vi "Delta_RT_manual_for_bigcryo.vi"() -> ()   [LabVIEW 2019]
uses:
  <vilib>/ptbypt/NI_PtbyPt.lvlib
panel:
  in  "Save R-H":bool
  in  "Measure R-H":bool
  in  "period [s]":dbl=0.5 caption="Delay Time (s)"
  out "R-H":cluster{"X":dbl[], "Y":dbl[]}[](graph) caption="XY Graph"
  in  "Reset R-H":bool
  in  "Period [s]":dbl=0.5 caption="Delay Time (s)"
  in  "Measure R-T":bool
  in  "Save R-T":bool
  out "R-T":cluster{"X":dbl[], "Y":dbl[]}[](graph) caption="XY Graph"
  out "Rate [K/min]":dbl=-0.03728307742891238 format="%#_6f"
  in  "Reset R-T":bool
  in  "Pause off":bool
  in  "Compliance [V]":dbl=1.0 format="%#_6f"
  out "VTI [K]":dbl=5.0082
  out "Delta Reading [Ohm]":dbl=1.19099581
  out "Sample Temp [K]":dbl=4.9552
  in  "Abort Delta":bool
  in  "Arm Delta":bool
  in  "DELAY [sec]":dbl=0.002 format="%#_6e"
  in  "I-HIGH [A]":dbl=0.0001 format="%#_6e"
  in  "Rate [K/min]":dbl=10.0
  in  "Set Temp [K]":dbl=1.0
  in  "Set Temperature":bool
  out "Magnetic Field [T]":dbl=-0.19938
  in  "Rate [T/min]":dbl=0.5
  in  "Set Field [T]":dbl=-0.2
  in  "Set Field":bool
  in  "Keithley":refnum<visa-resource-name>="GPIB1::20::INSTR"
  in  "Magnet Power supply":refnum<visa-resource-name>="COM7"
  in  "LakeShore350":refnum<visa-resource-name>="GPIB1::4::INSTR"
  out "error out 2":errorcluster={"status"=FALSE, "code"=1073676294, "source"="VISA Read in Delta_RT_manual_for_bigcryo.vi"}
  out "error out":errorcluster={"status"=FALSE, "code"=1073676294, "source"="VISA Read in Delta_RT_manual_for_bigcryo.vi"}
  # "Delta measurement"
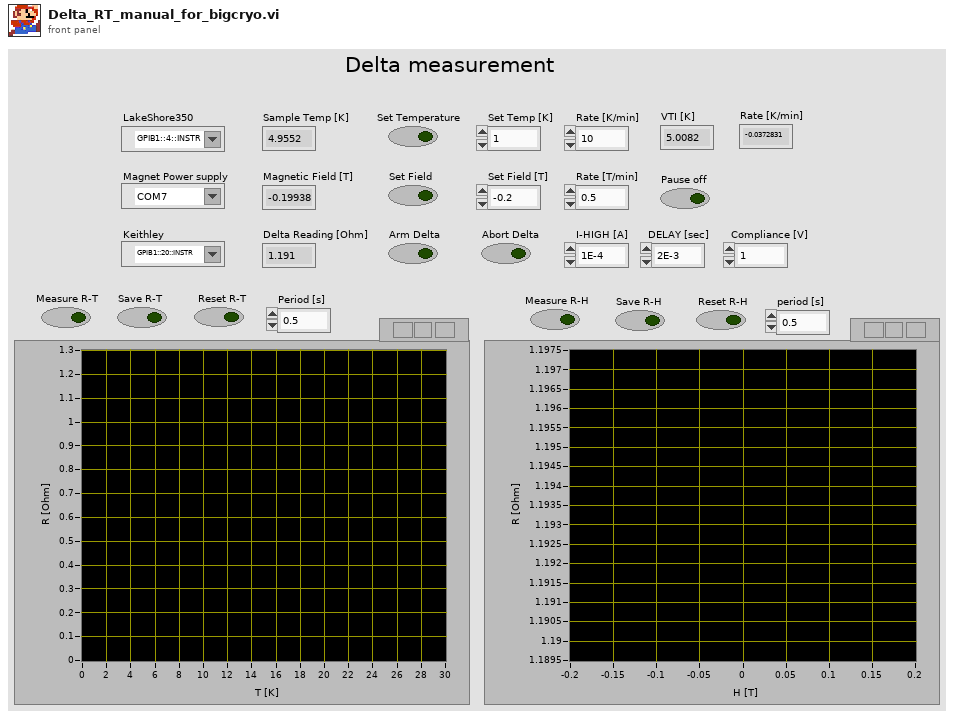
[diagram p1: front panel]
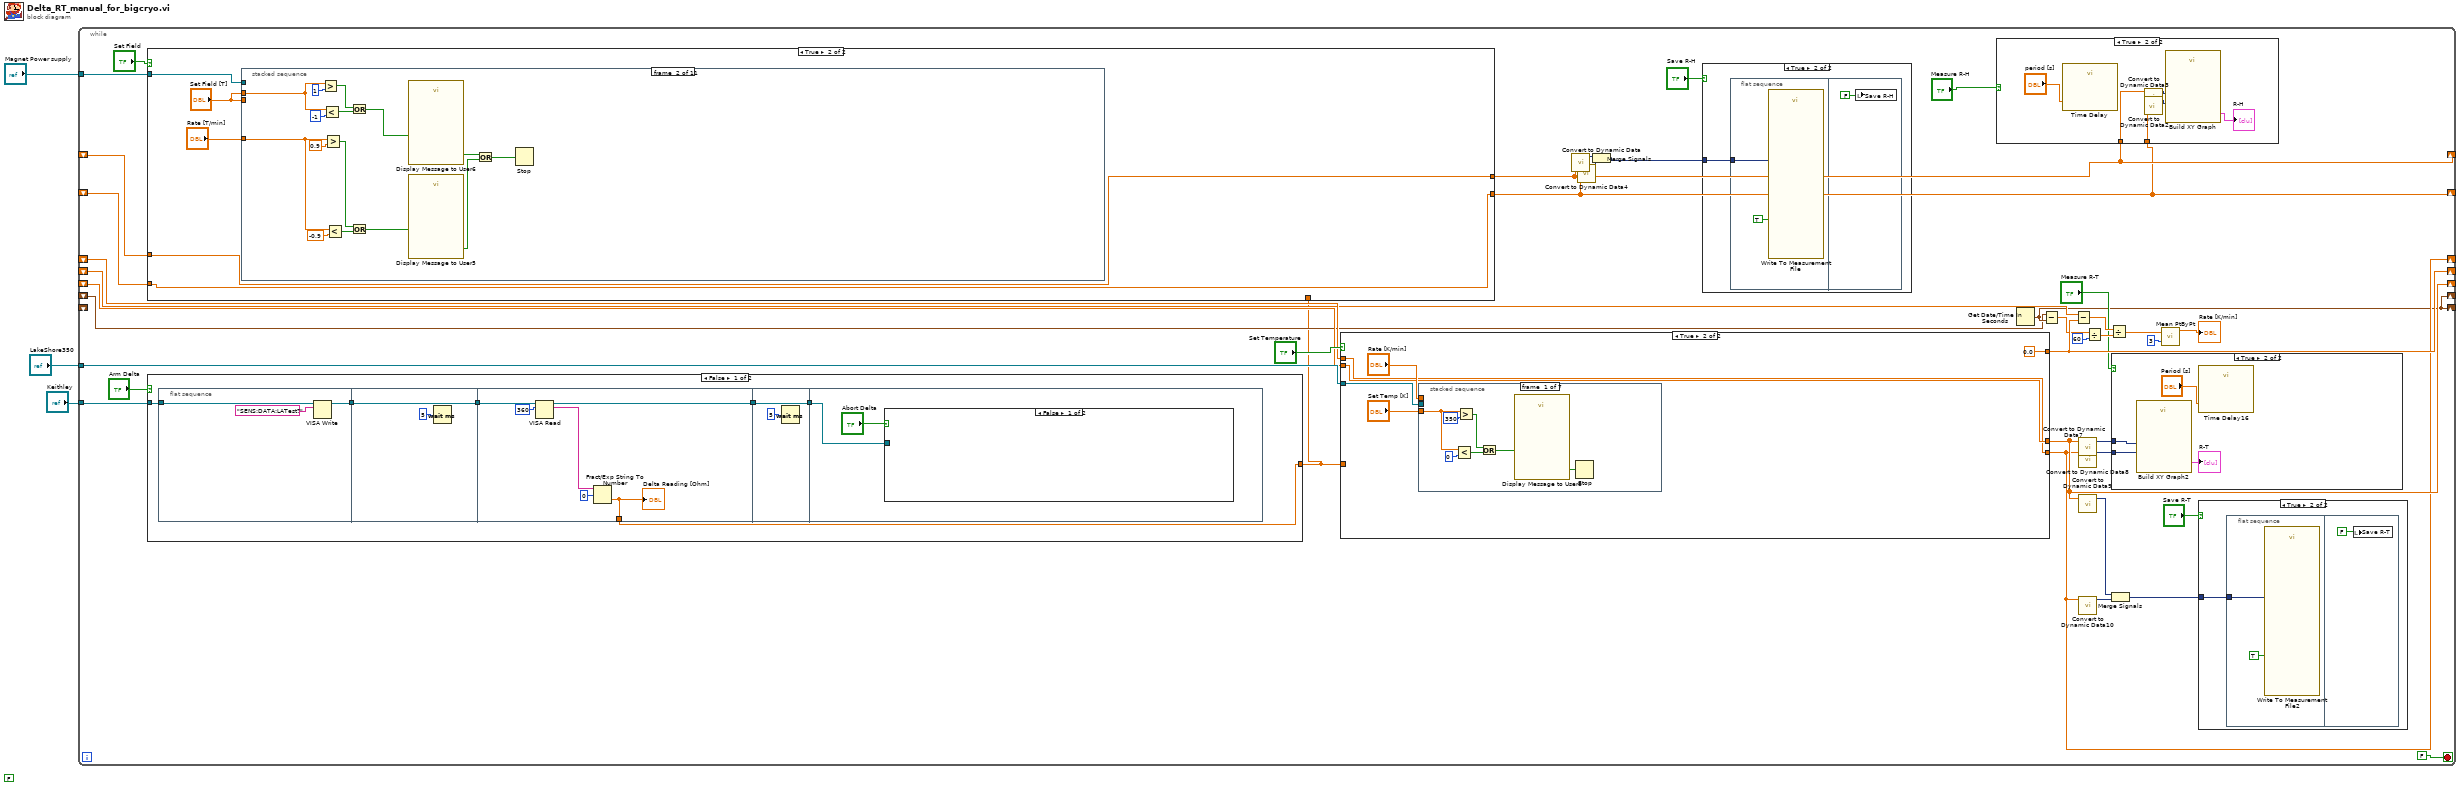
[diagram p0: block diagram]
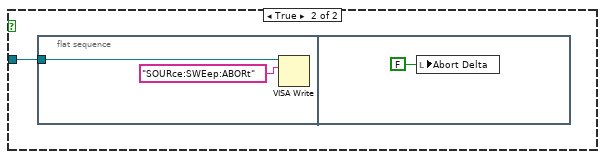
[diagram p6: hidden frame]
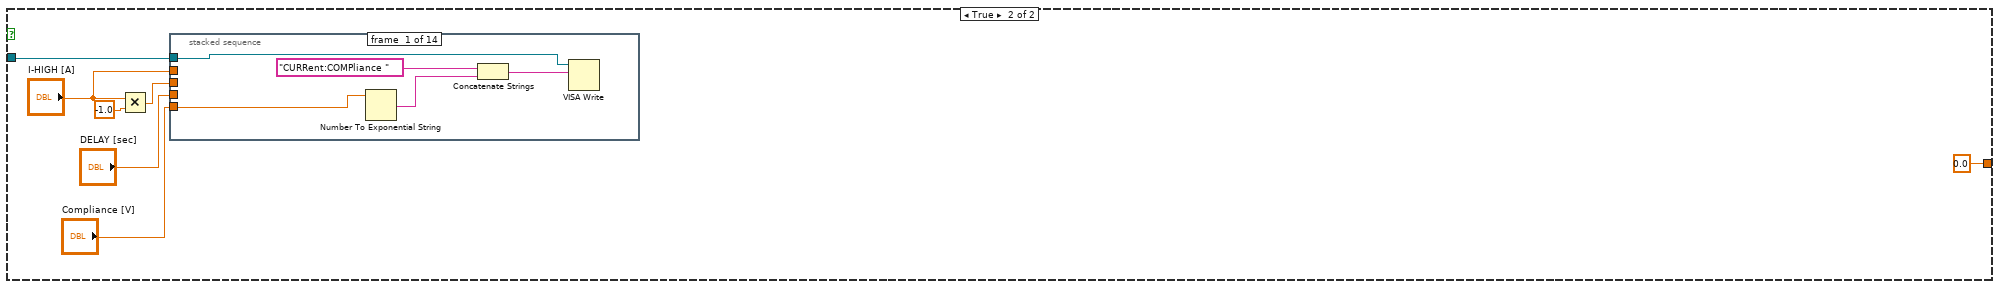
[diagram p7: hidden frame]
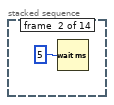
[diagram p8: hidden frame]
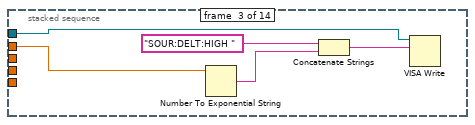
[diagram p9: hidden frame]
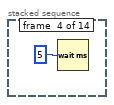
[diagram p10: hidden frame]
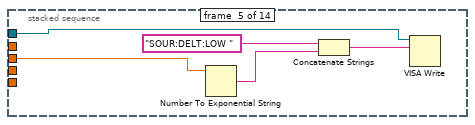
[diagram p11: hidden frame]
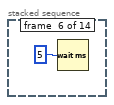
[diagram p12: hidden frame]
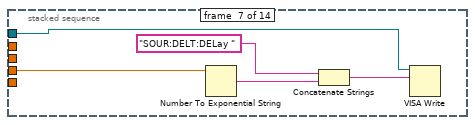
[diagram p13: hidden frame]
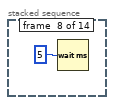
[diagram p14: hidden frame]
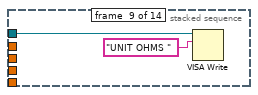
[diagram p15: hidden frame]
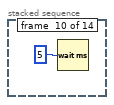
[diagram p16: hidden frame]
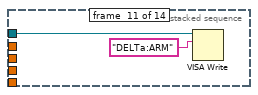
[diagram p17: hidden frame]
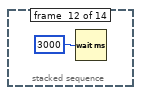
[diagram p18: hidden frame]
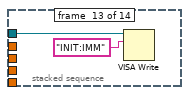
[diagram p19: hidden frame]
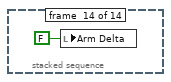
[diagram p20: hidden frame]
diagram:
  (unwired) FALSE
  n1 = while {
    tunnel: "Magnet Power supply" -> [w37]
    tunnel: "LakeShore350" -> [w40]
    tunnel: "Keithley" -> [w39]
    shift-right: [w26] -> _
    shift-left: _ -> [w21]
    shift-right: [w24] -> _
    shift-left: _ -> [w36]
    shift-right: [w19] -> _
    shift-left: _ -> [_]
    shift-right: [w34] -> _
    shift-left: _ -> [w35]
    shift-right: [w19] -> _
    shift-left: _ -> [w18]
    shift-right: [w7] -> _
    shift-left: _ -> [w12]
    shift-right: [w5] -> _
    shift-left: _ -> [w11]
    stop <- FALSE stop-if-true
    n2 = case shown="False" "Arm Delta" {
      tunnel: w39 -> [w66 w90]
      tunnel: [w61 0.0] -> w13
      frame False {
        n3 = flat-sequence {
          tunnel: w66 -> [w69]
          tunnel: [w67] -> w64
          tunnel: [w70] -> w65
          tunnel: w64 -> [w70]
          tunnel: w65 -> [w74]
          tunnel: [w73] -> w62
          tunnel: [w72] -> w61
          tunnel: [w78] -> w63
          tunnel: w62 -> [w78]
          tunnel: w63 -> [w80]
          frame #0 {
            n4 = VISA Write(VISA resource name=w69, write buffer="SENS:DATA:LATest?" ("write buffer 2")) -> (VISA resource name out=w67:refnum<visa-resource-name>)  [unwired: 1 in, 2 out]
          }
          frame #1 {
            n5 = Wait (ms)(milliseconds to wait=5) -> ()  [unwired: 1 out]
          }
          frame #2 {
            n6 = VISA Read(VISA resource name=w74, byte count=u32 360) -> (VISA resource name out=w73:refnum<visa-resource-name>, read buffer=w76:string)  [unwired: 1 in, 2 out]
            n7 = Fract/Exp String To Number(string=w76, offset=0) -> (number=w72:dbl)  [unwired: 3 out]
            "Delta Reading [Ohm]" <- w72
          }
          frame #3 {
            n8 = Wait (ms)(milliseconds to wait=5) -> ()  [unwired: 1 out]
          }
          frame #4 {
            n9 = case shown="False" "Abort Delta" {
              tunnel: w80 -> [_ w82]
              frame False {
              }
              frame True {
                n10 = flat-sequence {
                  tunnel: w82 -> [w84]
                  frame #0 {
                    n11 = VISA Write(VISA resource name=w84, write buffer="SOURce:SWEep:ABORt") -> ()  [unwired: 1 in, 3 out]
                  }
                  frame #1 {
                    n12 = local write "Abort Delta"(FALSE) -> ()
                  }
                }
              }
            }
          }
        }
      }
      frame True {
        n13 = Multiply(x="I-HIGH [A]", y=-1.0) -> (x*y=w89:dbl)
        n14 = stacked-sequence {
          tunnel: "I-HIGH [A]" -> [_ _ w101 _ _ _ _ _ _ _ _ _ _ _]
          tunnel: w90 -> [w94 _ w99 _ w106 _ w112 _ w117 _ w120 _ w123 _]
          tunnel: w89 -> [_ _ _ _ w105 _ _ _ _ _ _ _ _ _]
          tunnel: "DELAY [sec]" -> [_ _ _ _ _ _ w111 _ _ _ _ _ _ _]
          tunnel: "Compliance [V]" -> [w93 _ _ _ _ _ _ _ _ _ _ _ _ _]
          frame #0 {
            n15 = Number To Exponential String(number=w93) -> (E-format string=w96:string)  [unwired: 3 in]
            n16 = Concatenate Strings("CURRent:COMPliance ", w96) -> (w95:string)
            n17 = VISA Write(VISA resource name=w94, write buffer=w95) -> ()  [unwired: 1 in, 3 out]
          }
          frame #1 {
            n18 = Wait (ms)(milliseconds to wait=5) -> ()  [unwired: 1 out]
          }
          frame #2 {
            n19 = Number To Exponential String(number=w101) -> (E-format string=w102:string)  [unwired: 3 in]
            n20 = Concatenate Strings("SOUR:DELT:HIGH ", w102) -> (w100:string)
            n21 = VISA Write(VISA resource name=w99, write buffer=w100) -> ()  [unwired: 1 in, 3 out]
          }
          frame #3 {
            n22 = Wait (ms)(milliseconds to wait=5) -> ()  [unwired: 1 out]
          }
          frame #4 {
            n23 = Number To Exponential String(number=w105) -> (E-format string=w108:string)  [unwired: 3 in]
            n24 = Concatenate Strings("SOUR:DELT:LOW ", w108) -> (w107:string)
            n25 = VISA Write(VISA resource name=w106, write buffer=w107) -> ()  [unwired: 1 in, 3 out]
          }
          frame #5 {
            n26 = Wait (ms)(milliseconds to wait=5) -> ()  [unwired: 1 out]
          }
          frame #6 {
            n27 = Number To Exponential String(number=w111) -> (E-format string=w114:string)  [unwired: 3 in]
            n28 = Concatenate Strings("SOUR:DELT:DELay ", w114) -> (w113:string)
            n29 = VISA Write(VISA resource name=w112, write buffer=w113) -> ()  [unwired: 1 in, 3 out]
          }
          frame #7 {
            n30 = Wait (ms)(milliseconds to wait=5) -> ()  [unwired: 1 out]
          }
          frame #8 {
            n31 = VISA Write(VISA resource name=w117, write buffer="UNIT OHMS ") -> ()  [unwired: 1 in, 3 out]
          }
          frame #9 {
            n32 = Wait (ms)(milliseconds to wait=5) -> ()  [unwired: 1 out]
          }
          frame #10 {
            n33 = VISA Write(VISA resource name=w120, write buffer="DELTa:ARM") -> ()  [unwired: 1 in, 3 out]
          }
          frame #11 {
            n34 = Wait (ms)(milliseconds to wait=3000) -> ()  [unwired: 1 out]
          }
          frame #12 {
            n35 = VISA Write(VISA resource name=w123, write buffer="INIT:IMM") -> ()  [unwired: 1 in, 3 out]
          }
          frame #13 {
            n36 = local write "Arm Delta"(FALSE) -> ()
          }
        }
      }
    }
    n37 = case shown="True" "Set Field" {
      tunnel: w37 -> [w206 w289]
      tunnel: w13 -> [w204 _]
      tunnel: [w203 w288] -> w7
      tunnel: w12 -> [w202 w288]
      tunnel: [w201 w287] -> w5
      tunnel: w11 -> [w200 w287]
      frame False {
        n38 = stacked-sequence {
          seq-local: [w218 _ _ _ _ _ _ _] -> [_ w221 _ _ _ _ _ _]
          seq-local: [_ w219 _ _ _ _ _ _] -> [_ _ w225 _ _ _ _ _]
          seq-local: [_ w220 _ _ _ _ _ _] -> [_ _ w222 _ _ _ _ _]
          seq-local: [_ _ w224 _ _ _ _ _] -> [_ _ _ w265 _ _ _ _]
          seq-local: [_ _ w223 _ _ _ _ _] -> [_ _ _ w264 _ _ _ _]
          seq-local: [_ _ _ w267 _ _ _ _] -> [_ _ _ _ w270 _ _ _]
          seq-local: [_ _ _ w266 _ _ _ _] -> [_ _ _ _ w271 _ _ _]
          seq-local: [_ _ _ _ w270 _ _ _] -> [_ _ _ _ _ w282 _ _]
          seq-local: [_ _ _ _ w271 _ _ _] -> [_ _ _ _ _ w280 _ _]
          seq-local: [_ _ _ _ _ w281 _ _] -> [_ _ _ _ _ _ _ w286]
          seq-local: [_ _ _ _ _ w279 _ _] -> [_ _ _ _ _ _ _ w285]
          tunnel: w206 -> [w218 _ _ _ _ _ _ _]
          tunnel: [_ _ _ _ _ w272 _ _] -> w205
          frame #0 {
          }
          frame #1 {
            n39 = VISA Clear(VISA resource name=w221) -> (VISA resource name out=w219:refnum<visa-resource-name>, error out=w220:errorcluster)  [unwired: 1 in]
          }
          frame #2 {
            n40 = flat-sequence {
              tunnel: w225 -> [w229]
              tunnel: [w228] -> w224
              tunnel: [w227] -> w223
              tunnel: w222 -> [w226]
              frame #0 {
                n41 = call "Time Delay8"() -> ()  [unwired: 11 in, 1 out]
              }
              frame #1 {
                n42 = case shown="False" "Pause off" {
                  tunnel: w229 -> [w232 w244]
                  tunnel: [w232 w233] -> w228
                  tunnel: [w231 w236] -> w227
                  tunnel: w226 -> [w231 w239]
                  frame False {
                  }
                  frame True {
                    n43 = flat-sequence {
                      tunnel: w244 -> [w248]
                      tunnel: [w247] -> w242
                      tunnel: [w246] -> w240
                      tunnel: w239 -> [w245]
                      tunnel: [w253] -> w243
                      tunnel: w242 -> [w253]
                      tunnel: [w252] -> w241
                      tunnel: w240 -> [w252]
                      tunnel: w243 -> [w255]
                      tunnel: w241 -> [_]
                      tunnel: [w255] -> w238
                      tunnel: [w254] -> w234
                      tunnel: w238 -> [w257]
                      tunnel: [w257] -> w237
                      tunnel: [w256] -> w235
                      tunnel: w234 -> [w256]
                      tunnel: [w261] -> w233
                      tunnel: w237 -> [w260]
                      tunnel: [w259] -> w236
                      tunnel: w235 -> [w258]
                      frame #0 {
                        n44 = Concatenate Strings("P 0" ("Command"), "\r") -> (w250:string)
                        n45 = VISA Write(VISA resource name=w248, write buffer=w250, error in (no error)=w245) -> (VISA resource name out=w247:refnum<visa-resource-name>, error out=w246:errorcluster)  [unwired: 1 out]
                      }
                      frame #1 {
                        n46 = call "Time Delay14"() -> ()  [unwired: 11 in, 1 out]
                      }
                      frame #2 {
                        n47 = VISA Close(VISA resource name=w255) -> (error out=w254:errorcluster)  [unwired: 1 in]
                      }
                      frame #3 {
                        n48 = call "Time Delay15"() -> ()  [unwired: 11 in, 1 out]
                      }
                      frame #4 {
                        n49 = VISA Clear(VISA resource name=w260, error in (no error)=w258) -> (VISA resource name out=w261:refnum<visa-resource-name>, error out=w259:errorcluster)
                      }
                      frame #5 {
                        n50 = local write "Pause off"(FALSE) -> ()
                      }
                    }
                  }
                }
              }
            }
          }
          frame #3 {
            n51 = Concatenate Strings("G O" ("Command"), "\r") -> (w268:string)
            n52 = VISA Write(VISA resource name=w265, write buffer=w268, error in (no error)=w264) -> (VISA resource name out=w267:refnum<visa-resource-name>, error out=w266:errorcluster)  [unwired: 1 out]
          }
          frame #4 {
            n53 = call "Time Delay9"() -> ()  [unwired: 11 in, 1 out]
          }
          frame #5 {
            n54 = VISA Read(VISA resource name=w282, byte count=u32 30, error in (no error)=w280) -> (VISA resource name out=w281:refnum<visa-resource-name>, read buffer=w276:string, error out=w279:errorcluster)  [unwired: 1 out]
            n55 = Match Pattern(string=w276, regular expression="OUTPUT:") -> (after substring=w274:string)  [unwired: 1 in, 3 out]
            n56 = Match Pattern(string=w274, regular expression=" TESLA") -> (before substring=w273:string)  [unwired: 1 in, 3 out]
            n57 = Fract/Exp String To Number(string=w273, offset=0) -> (number=w272:dbl)  [unwired: 2 in, 1 out]
          }
          frame #6 {
            n58 = call "Time Delay10"() -> ()  [unwired: 11 in, 1 out]
          }
          frame #7 {
            n59 = VISA Close(VISA resource name=w286, error in (no error)=w285) -> (error out=→"error out":errorcluster)
          }
        }
        "Magnetic Field [T]" <- w205
        n60 = case shown="False" "Reset R-H" {
          tunnel: w205 -> [w212 _]
          tunnel: [w211 w214] -> w203
          tunnel: [w210 w213] -> w201
          tunnel: w204 -> [w209 _]
          tunnel: w202 -> [w208 _]
          tunnel: w200 -> [w207 _]
          frame False {
            n61 = Build Array (concatenate)(w208, w212) -> (w211:dbl[])
            n62 = Build Array (concatenate)(w207, w209) -> (w210:dbl[])
          }
          frame True {
            n63 = stacked-sequence {
              tunnel: [dbl[] [] _] -> w214
              tunnel: [dbl[] [] _] -> w213
              frame #0 {
              }
              frame #1 {
                n64 = local write "Reset R-H"(FALSE) -> ()
              }
            }
          }
        }
      }
      frame True {
        n65 = stacked-sequence {
          tunnel: w289 -> [w292 _ _ w311 _ w356 _ w374 _ w379 _]
          tunnel: "Set Field [T]" -> [_ w294 _ _ _ _ _ _ _ _ _]
          tunnel: "Rate [T/min]" -> [_ w293 _ _ _ _ _ w364 _ _ _]
          tunnel: "Set Field [T]" -> [_ _ _ w310 _ w354 _ _ _ _ _]
          frame #0 {
            n66 = VISA Clear(VISA resource name=w292) -> ()  [unwired: 1 in, 2 out]
          }
          frame #1 {
            n67 = Greater?(x=w294, y=1) -> (0:w295:bool)
            n68 = Less?(x=w294, y=-1) -> (x < y?=w300:bool)
            n69 = Greater?(x=w293, y=0.9) -> (0:w304:bool)
            n70 = Less?(x=w293, y=-0.9) -> (x < y?=w303:bool)
            n71 = Or(x=w295, y=w300) -> (x .or. y?=w306:bool)
            n72 = Or(x=w304, y=w303) -> (x .or. y?=w305:bool)
            n73 = call "Display Message to User6"("Enable"=w306) -> ("OK"=w307:bool)  [unwired: 9 in, 1 out]
            n74 = call "Display Message to User5"("Enable"=w305) -> ("OK"=w296:bool)  [unwired: 9 in, 1 out]
            n75 = Or(x=w307, y=w296) -> (x .or. y?=w297:bool)
            n76 = Stop(stop? (T)=w297) -> ()
          }
          frame #2 {
            n77 = Wait (ms)(milliseconds to wait=500) -> ()  [unwired: 1 out]
          }
          frame #3 {
            # "Read Magnetic Field"
            # "for safety"
            # "polarity"
            n78 = stacked-sequence {
              seq-local: [w315 _ _ _ _ _ _ _] -> [_ w318 _ _ _ _ _ _]
              seq-local: [_ w316 _ _ _ _ _ _] -> [_ _ w320 _ _ _ _ _]
              seq-local: [_ w317 _ _ _ _ _ _] -> [_ _ w319 _ _ _ _ _]
              seq-local: [_ _ w320 _ _ _ _ _] -> [_ _ _ w323 _ _ _ _]
              seq-local: [_ _ w319 _ _ _ _ _] -> [_ _ _ w322 _ _ _ _]
              seq-local: [_ _ _ w325 _ _ _ _] -> [_ _ _ _ w328 _ _ _]
              seq-local: [_ _ _ w324 _ _ _ _] -> [_ _ _ _ w329 _ _ _]
              seq-local: [_ _ _ _ w328 _ _ _] -> [_ _ _ _ _ w340 _ _]
              seq-local: [_ _ _ _ w329 _ _ _] -> [_ _ _ _ _ w338 _ _]
              seq-local: [_ _ _ _ _ w339 _ _] -> [_ _ _ _ _ _ _ w344]
              seq-local: [_ _ _ _ _ w337 _ _] -> [_ _ _ _ _ _ _ w343]
              tunnel: w311 -> [w315 _ _ _ _ _ _ _]
              tunnel: [_ _ _ _ _ w330 _ _] -> w312
              frame #0 {
              }
              frame #1 {
                n79 = VISA Clear(VISA resource name=w318) -> (VISA resource name out=w316:refnum<visa-resource-name>, error out=w317:errorcluster)  [unwired: 1 in]
              }
              frame #2 {
                n80 = call "Time Delay6"() -> ()  [unwired: 11 in, 1 out]
              }
              frame #3 {
                n81 = Concatenate Strings("G O" ("Command"), "\r") -> (w326:string)
                n82 = VISA Write(VISA resource name=w323, write buffer=w326, error in (no error)=w322) -> (VISA resource name out=w325:refnum<visa-resource-name>, error out=w324:errorcluster)  [unwired: 1 out]
              }
              frame #4 {
                n83 = call "Time Delay7"() -> ()  [unwired: 11 in, 1 out]
              }
              frame #5 {
                n84 = VISA Read(VISA resource name=w340, byte count=u32 30, error in (no error)=w338) -> (VISA resource name out=w339:refnum<visa-resource-name>, read buffer=w334:string, error out=w337:errorcluster)  [unwired: 1 out]
                n85 = Match Pattern(string=w334, regular expression="OUTPUT:") -> (after substring=w332:string)  [unwired: 1 in, 3 out]
                n86 = Match Pattern(string=w332, regular expression=" TESLA") -> (before substring=w331:string)  [unwired: 1 in, 3 out]
                n87 = Fract/Exp String To Number(string=w331, offset=0) -> (number=w330:dbl)  [unwired: 2 in, 1 out]
              }
              frame #6 {
                n88 = call "Time Delay11"() -> ()  [unwired: 11 in, 1 out]
              }
              frame #7 {
                n89 = VISA Close(VISA resource name=w344, error in (no error)=w343) -> (error out=→"error out 2":errorcluster)
              }
            }
            n90 = Absolute Value(x=w312) -> (abs(x)=w313:dbl)
            n91 = Less?(x=w313, y=0.002) -> (x < y?=w309:bool)
            n92 = case shown="True" w309 {
              tunnel: w311 -> [_ w347]
              tunnel: w310 -> [_ w345]
              frame False {
              }
              frame True {
                n93 = Greater Or Equal To 0?(x=w345) -> (x >= 0?=w346:bool)
                n94 = case shown="True" w346 {
                  tunnel: ["D [-]" ("data") "D [+]" ("data")] -> w348
                  frame False {
                  }
                  frame True {
                  }
                }
                n95 = Concatenate Strings(w348, "\r") -> (w350:string)
                n96 = VISA Write(VISA resource name=w347, write buffer=w350) -> ()  [unwired: 1 in, 3 out]
              }
            }
          }
          frame #4 {
            n97 = Wait (ms)(milliseconds to wait=500) -> ()  [unwired: 1 out]
          }
          frame #5 {
            # "set set field"
            n98 = Number To Fractional String(number=w354, width (-)=i16 6, precision (6)=i16 3) -> (F-format string=w359:string)  [unwired: 1 in]
            n99 = Concatenate Strings("S [%][MID] " ("string"), w359) -> (w355:string)
            n100 = Concatenate Strings(w355, "\r") -> (w358:string)
            n101 = VISA Write(VISA resource name=w356, write buffer=w358) -> ()  [unwired: 1 in, 3 out]
          }
          frame #6 {
            n102 = Wait (ms)(milliseconds to wait=500) -> ()  [unwired: 1 out]
          }
          frame #7 {
            # "set rate"
            n103 = Divide(x=w364, y=60.0) -> (x/y=w369:dbl)
            n104 = Divide(x=w369, y=0.09797) -> (x/y=w367:dbl)
            n105 = Number To Fractional String(number=w367, width (-)=i16 6, precision (6)=i16 3) -> (F-format string=w372:string)  [unwired: 1 in]
            n106 = Concatenate Strings("S R " ("string"), w372) -> (w371:string)
            n107 = Concatenate Strings(w371, "\r") -> (w376:string)
            n108 = VISA Write(VISA resource name=w374, write buffer=w376) -> ()  [unwired: 1 in, 3 out]
          }
          frame #8 {
            n109 = Wait (ms)(milliseconds to wait=500) -> ()  [unwired: 1 out]
          }
          frame #9 {
            # "Go to set field"
            n110 = Concatenate Strings("R [%][MID]" ("data"), "\r") -> (w381:string)
            n111 = VISA Write(VISA resource name=w379, write buffer=w381) -> ()  [unwired: 1 in, 3 out]
          }
          frame #10 {
            n112 = local write "Set Field"(FALSE) -> ()
            n113 = Wait (ms)(milliseconds to wait=500) -> ()  [unwired: 1 out]
          }
        }
      }
    }
    n114 = case shown="True" "Set Temperature" {
      tunnel: w40 -> [w136 w172]
      tunnel: [w131 w169] -> w26
      tunnel: w21 -> [w132 w169]
      tunnel: w13 -> [w130 _]
      tunnel: [w129 w168] -> w24
      tunnel: w36 -> [w128 w168]
      tunnel: [w126 0.0] -> w34
      frame False {
        n115 = flat-sequence {
          tunnel: w136 -> [w150]
          tunnel: [w149] -> w134
          tunnel: [w148] -> w133
          tunnel: [w148] -> w126
          tunnel: [w157] -> w135
          tunnel: w134 -> [w157]
          tunnel: w135 -> [w159]
          frame #0 {
            n116 = Concatenate Strings("KRDG?B" ("write buffer"), "\n") -> (w155:string)
            n117 = VISA Write(VISA resource name=w150, write buffer=w155) -> (VISA resource name out=w153:refnum<visa-resource-name>)  [unwired: 1 in, 2 out]
            n118 = VISA Read(VISA resource name=w153, byte count=u32 100) -> (VISA resource name out=w149:refnum<visa-resource-name>, read buffer=w151:string)  [unwired: 1 in, 2 out]
            n119 = Fract/Exp String To Number(string=w151) -> (number=w148:dbl)  [unwired: 3 in, 1 out]
            "Sample Temp [K]" <- w148
          }
          frame #1 {
            n120 = Wait (ms)(milliseconds to wait=5) -> ()  [unwired: 1 out]
          }
          frame #2 {
            n121 = Concatenate Strings("KRDG?A" ("write buffer"), "\n") -> (w165:string)
            n122 = VISA Write(VISA resource name=w159, write buffer=w165) -> (VISA resource name out=w163:refnum<visa-resource-name>)  [unwired: 1 in, 2 out]
            n123 = VISA Read(VISA resource name=w163, byte count=u32 100) -> (read buffer=w161:string)  [unwired: 1 in, 3 out]
            n124 = Fract/Exp String To Number(string=w161) -> (number=→"VTI [K]":dbl)  [unwired: 3 in, 1 out]
          }
        }
        n125 = case shown="False" "Reset R-T" {
          tunnel: w133 -> [w142 _]
          tunnel: w132 -> [w141 _]
          tunnel: [w140 w144] -> w131
          tunnel: w130 -> [w139 _]
          tunnel: [w138 w143] -> w129
          tunnel: w128 -> [w137 _]
          frame False {
            n126 = Build Array (concatenate)(w141, w142) -> (w140:dbl[])
            n127 = Build Array (concatenate)(w137, w139) -> (w138:dbl[])
          }
          frame True {
            n128 = stacked-sequence {
              tunnel: [dbl[] [] _] -> w144
              tunnel: [dbl[] [] _] -> w143
              frame #0 {
              }
              frame #1 {
                n129 = local write "Reset R-T"(FALSE) -> ()
              }
            }
          }
        }
      }
      frame True {
        n130 = stacked-sequence {
          tunnel: w172 -> [_ w180 _ w187 _ w194 _]
          tunnel: "Set Temp [K]" -> [w174 _ _ _ _ w192 _]
          tunnel: "Rate [K/min]" -> [_ _ _ w186 _ _ _]
          frame #0 {
            n131 = Less?(x=w174, y=0) -> (x < y?=w178:bool)
            n132 = Greater?(x=w174, y=350) -> (0:w175:bool)
            n133 = Or(x=w175, y=w178) -> (x .or. y?=w179:bool)
            n134 = call "Display Message to User8"("Enable"=w179) -> ("OK"=w173:bool)  [unwired: 9 in, 1 out]
            n135 = Stop(stop? (T)=w173) -> ()
          }
          frame #1 {
            n136 = Concatenate Strings("OUTMODE 1, 1, 2, 1" ("write buffer"), "\n") -> (w181:string)
            n137 = VISA Write(VISA resource name=w180, write buffer=w181) -> ()  [unwired: 1 in, 3 out]
          }
          frame #2 {
            n138 = Wait (ms)(milliseconds to wait=u32 50) -> ()  [unwired: 1 out]
          }
          frame #3 {
            n139 = Number To Fractional String(number=w186) -> (F-format string=w185:string)  [unwired: 3 in]
            n140 = Concatenate Strings("RAMP 1, 1," ("write buffer"), w185, "\n") -> (w189:string)
            n141 = VISA Write(VISA resource name=w187, write buffer=w189) -> ()  [unwired: 1 in, 3 out]
          }
          frame #4 {
            n142 = Wait (ms)(milliseconds to wait=u32 50) -> ()  [unwired: 1 out]
          }
          frame #5 {
            n143 = Number To Fractional String(number=w192) -> (F-format string=w193:string)  [unwired: 3 in]
            n144 = Concatenate Strings("SETP 1," ("write buffer"), w193, "\n") -> (w196:string)
            n145 = VISA Write(VISA resource name=w194, write buffer=w196) -> ()  [unwired: 1 in, 3 out]
          }
          frame #6 {
            n146 = local write "Set Temperature"(FALSE) -> ()
          }
        }
      }
    }
    n147 = call "Convert to Dynamic Data"("Array"=w7) -> ("Dynamic Data Type"=w6:dynamicdata)  [unwired: 3 in]
    n148 = call "Convert to Dynamic Data4"("Array"=w5) -> ("Dynamic Data Type"=w4:dynamicdata)  [unwired: 3 in]
    n149 = Merge Signals(w6, w4) -> (w8:dynamicdata)
    n150 = case shown="True" "Save R-H" {
      tunnel: w8 -> [_ w43]
      frame False {
      }
      frame True {
        n151 = flat-sequence {
          tunnel: w43 -> [w44]
          frame #0 {
            n152 = call "Write To Measurement File"("Signals"=w44, "Reset"=TRUE) -> ()  [unwired: 15 in, 3 out]
          }
          frame #1 {
            n153 = local write "Save R-H"(FALSE) -> ()
          }
        }
      }
    }
    n154 = case shown="True" "Measure R-H" {
      tunnel: w5 -> [_ w51]
      tunnel: w7 -> [_ w49]
      frame False {
      }
      frame True {
        n155 = call "Time Delay"("Delay Time (s)"="period [s]") -> ()  [unwired: 10 in, 1 out]
        n156 = call "Convert to Dynamic Data3"("Array"=w49) -> ("Dynamic Data Type"=w48:dynamicdata)  [unwired: 3 in]
        n157 = call "Convert to Dynamic Data2"("Array"=w51) -> ("Dynamic Data Type"=w50:dynamicdata)  [unwired: 3 in]
        n158 = call "Build XY Graph"("Y Input"=w50, "X Input"=w48) -> ("XY Graph"=→"R-H":cluster{"X":dbl[], "Y":dbl[]}[])  [unwired: 8 in, 1 out]
      }
    }
    n159 = Get Date/Time In Seconds() -> (seconds since 1Jan1904=w19:timestamp)
    n160 = Subtract(x=w18, y=w19) -> (x-y=w33:dbl)
    n161 = Subtract(x=w35, y=w34) -> (x-y=w30:dbl)
    n162 = call "Convert to Dynamic Data7"("Array"=w26) -> ("Dynamic Data Type"=w29:dynamicdata)  [unwired: 3 in]
    n163 = call "Convert to Dynamic Data8"("Array"=w24) -> ("Dynamic Data Type"=w28:dynamicdata)  [unwired: 3 in]
    n164 = call "Convert to Dynamic Data9"("Array"=w26) -> ("Dynamic Data Type"=w25:dynamicdata)  [unwired: 3 in]
    n165 = call "Convert to Dynamic Data10"("Array"=w24) -> ("Dynamic Data Type"=w23:dynamicdata)  [unwired: 3 in]
    n166 = Divide(x=w33, y=60) -> (x/y=w31:dbl)
    n167 = Divide(x=w30, y=w31) -> (x/y=w16:dbl)
    n168 = case shown="True" "Measure R-T" {
      tunnel: w29 -> [_ w56]
      tunnel: w28 -> [_ w53]
      frame False {
      }
      frame True {
        n169 = call "Build XY Graph2"("Y Input"=w53, "X Input"=w56) -> ("XY Graph"=→"R-T":cluster{"X":dbl[], "Y":dbl[]}[])  [unwired: 8 in, 1 out]
        n170 = call "Time Delay16"("Delay Time (s)"="Period [s]") -> ()  [unwired: 10 in, 1 out]
      }
    }
    n171 = Merge Signals(w25, w23) -> (w27:dynamicdata)
    n172 = call <vilib>:"Mean PtByPt.vi"("x"=w16, "sample length"=3) -> ("mean"=→"Rate [K/min]":dbl)  [unwired: 2 in, 1 out]
    n173 = case shown="True" "Save R-T" {
      tunnel: w27 -> [_ w57]
      frame False {
      }
      frame True {
        n174 = flat-sequence {
          tunnel: w57 -> [w58]
          frame #0 {
            n175 = call "Write To Measurement File2"("Signals"=w58, "Reset"=TRUE) -> ()  [unwired: 15 in, 3 out]
          }
          frame #1 {
            n176 = local write "Save R-T"(FALSE) -> ()
          }
        }
      }
    }
  }
